vi "Inspect osq.vi"() -> ()   [LabVIEW 2013]
uses:
  Tools/Line.ctl
  <vilib>/Analysis/polynomials.llb/Unique Numbers and Multiplicity (DBL).vi
  <vilib>/Analysis/NI_AALPro.lvlib
panel:
  in  "Open (*.osq)":path=path "C:/Users/Adam/Documents/h5seq/Examples/acquire.osq"
  in  "Tab Control":enum32{"Plot", "VARS"}(tab)
  out "Waveform Graph":dbl[][](graph)=[[10.0, 20.0, 30.0, 40.0, 50.0, 60.0, 70.0, 80.0, 90.0, 100.0], [10.0, 20.0, 30.0, 40.0, 50.0, 60.0, 70.0, 80.0, 90.0, 100.0]]
  in  "VAR":u16(ring) items=["ACQ"]
  out "min":dbl=10.0
  out "max":dbl=100.0
  out "Number":i32=10
  out "Unique":i32=10
  out "Step size (average)":dbl=10.0
  out "VARS":string[](array[string])=["ACQ"]
  out "SEQs":T1[](array[typedef])=[{"Var Array"=[["ACQ", "10"]], "Comment"=""}, {"Var Array"=[["ACQ", "20"]], "Comment"=""}, {"Var Array"=[["ACQ", "30"]], "Comment"=""}, {"Var Array"=[["ACQ", "40"]], "Comment"=""}, {"Var Array"=[["ACQ", "50"]], "Comment"=""}, {"Var Array"=[["ACQ", "60"]], "Comment"=""}, {"Var Array"=[["ACQ", "70"]], "Comment"=""}, {"Var Array"=[["ACQ", "80"]], "Comment"=""}, {"Var Array"=[["ACQ", "90"]], "Comment"=""}, {"Var Array"=[["ACQ", "100"]], "Comment"=""}]
  in  "stop":bool
  # "Inspect"
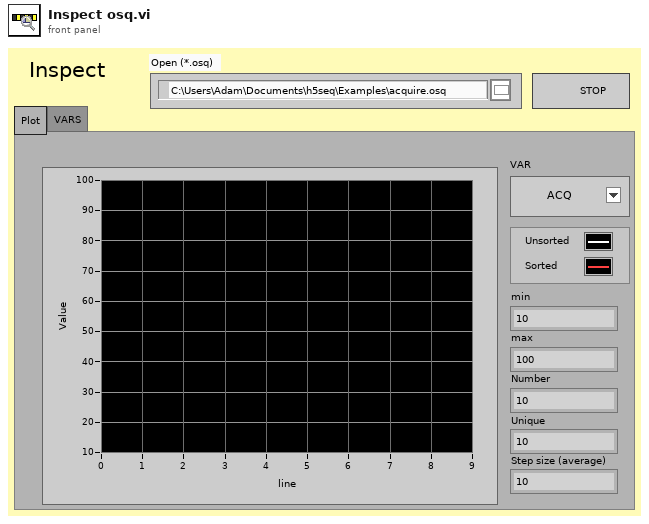
[diagram p1: front panel]
types:
  T1 = typedef "Line.ctl" = cluster{"Var Array":string[][], "Comment":string}
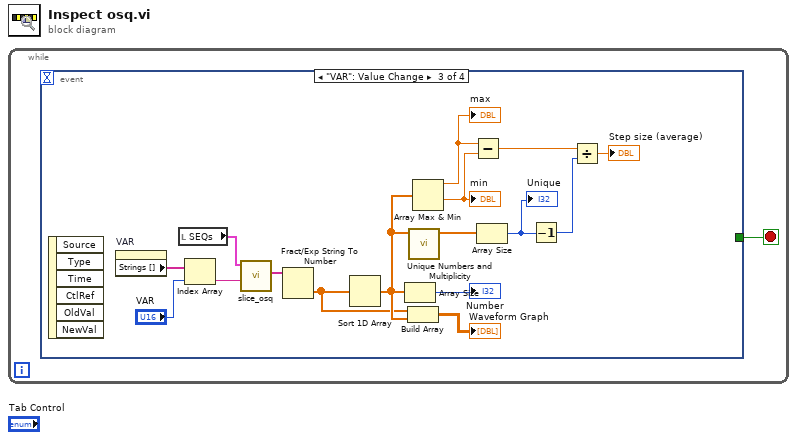
[diagram p0: block diagram]
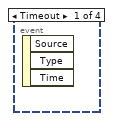
[diagram p2: hidden frame]
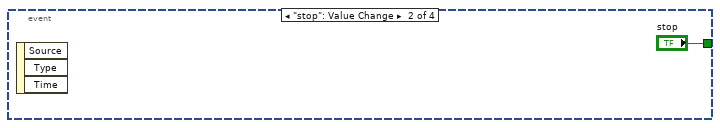
[diagram p3: hidden frame]
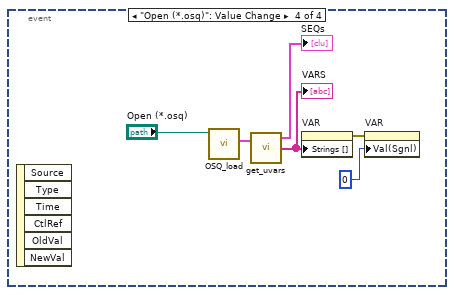
[diagram p4: hidden frame]
diagram:
  n1 = while {
    stop <- w1 stop-if-true
    n2 = event shown="[2] \"VAR\": Value Change" {
      selector: _ -> [_ _ _ _]
      dyn-events: _ -> [_ _ _ _]
      timeout: _ -> [_ _ _ _]
      tunnel: [_ "stop" _ _] -> w1
      event Timeout {
        n3 = event-data() -> ()  [unwired: 1 in, 3 out]
      }
      event "stop": Value Change {
        n4 = event-data() -> ()  [unwired: 1 in, 3 out]
      }
      event "VAR": Value Change {
        n5 = event-data() -> ()  [unwired: 1 in, 6 out]
        n6 = property on="VAR" class="Ring (strict)"() -> ("Strings []"=w6:string[])  [unwired: 2 in, 2 out]
        n7 = local read "SEQs"() -> (w7:T1[])
        n8 = Index Array(array=w6, index="VAR") -> (element=w4:string)
        n9 = call "slice_osq.vi"("VAR"=w4, "SEQs in"=w7) -> ("VALS"=w3:string[])  [unwired: 8 in, 1 out]
        n10 = Fract/Exp String To Number(string=w3) -> (number=w8:dbl[])  [unwired: 3 in, 1 out]
        n11 = Sort 1D Array(array=w8) -> (sorted array=w13:dbl[])
        n12 = Array Size(array=w13) -> (size(s)=→"Number":i32)
        n13 = Build Array(w8, w13) -> (→"Waveform Graph":dbl[][])
        n14 = call-poly <vilib>:"Unique Numbers and Multiplicity.vi"("Numbers"=w13) -> ("Unique Numbers"=w12:dbl[])  [unwired: 8 in, 2 out]
        n15 = Array Max & Min(array=w13) -> (max value=w17:dbl, min value=w11:dbl)  [unwired: 2 out]
        "max" <- w17
        "min" <- w11
        n16 = Subtract(x=w17, y=w11) -> (x-y=w16:dbl)
        n17 = Array Size(array=w12) -> (size(s)=w10:i32)
        "Unique" <- w10
        n18 = Decrement(x=w10) -> (x-1=w9:i32)
        n19 = Divide(x=w16, y=w9) -> (x/y=→"Step size (average)":dbl)
      }
      event "Open (*.osq)": Value Change {
        n20 = event-data() -> ()  [unwired: 1 in, 6 out]
        n21 = call "OSQ_load.vi"("Open"="Open (*.osq)") -> ("SEQs"=w21:T1[])  [unwired: 7 in, 3 out]
        n22 = call "get_uvars.vi"("SEQs in"=w21) -> ("SEQs out"=→"SEQs":T1[], "UVARS"=w20:string[])  [unwired: 1 in, 1 out]
        "VARS" <- w20
        n23 = property on="VAR" class="Ring (strict)"("Strings []"=w20) -> (error out=w23:errorcluster)  [unwired: 2 in, 1 out]
        n24 = property on="VAR" class="Ring (strict)"(error in=w23, "Val(Sgnl)"=u16 0 ("Value (Signaling)")) -> ()  [unwired: 1 in, 2 out]
      }
    }
  }
